vi "SRV_Check-Establish Directory Path.vi"(8 "error in (no error)":errorcluster, 11 "Directory Path":path) -> (0 "error out":errorcluster, 3 "Directory Path dup":path)   [LabVIEW 2014]
doc: "Checks to see if Directory Path exists. If it does not exist, the VI will attempt to create it. An error will be returned if not successful.\n\n\nAuthor: Mike Schultz"
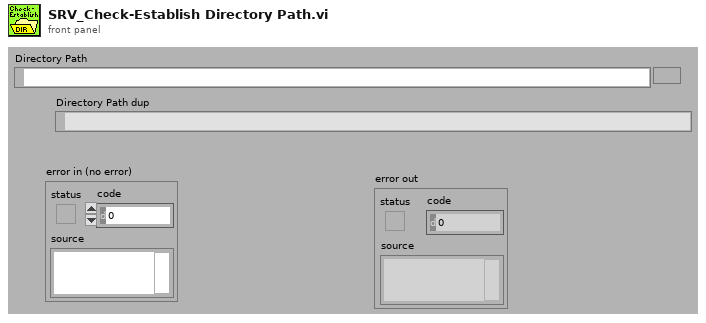
[diagram p1: front panel]
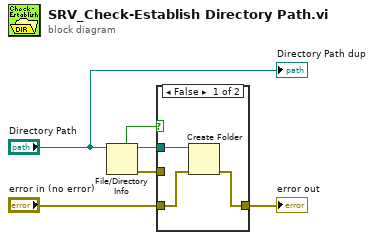
[diagram p0: block diagram]
diagram:
  n1 = File/Directory Info(path="Directory Path") -> (path out=w6:path, directory=w5:bool, error out=w1:errorcluster)  [unwired: 1 in, 4 out]
  n2 = case shown="False" w5 {
    tunnel: w6 -> [w9 _]
    tunnel: "error in (no error)" -> [w8 w10]
    tunnel: [w7 w10] -> w3
    tunnel: w1 -> [_ _]
    frame False {
      n3 = Create Folder(path (use dialog)=w9, error in=w8) -> (error out=w7:errorcluster)  [unwired: 1 in, 2 out]
    }
    frame True {
    }
  }
  "error out" <- w3
  "Directory Path dup" <- "Directory Path"
